vi "Top.vi"(8 "error in (no error)":errorcluster, 11 "Thread in":refnum<class "Thread.lvclass">) -> (0 "error":errorcluster, 3 "Thread out":refnum<class "Thread.lvclass">)   [LabVIEW 2017, in "DSF Core.lvlib" / "Thread.lvclass"]
uses:
  Thread.lvclass
  Thread State.ctl
  Thread.lvclass/Thread.ctl
  Thread Parameters/Thread Parameters.lvclass/Thread Parameters.ctl
  <vilib>/Platform/TimedLoop/XDataNode/timing_clust.ctl
  <vilib>/Platform/TimedLoop/XDataNode/nitl_modes.ctl
  <vilib>/Platform/TimedLoop/XDataNode/wakeup.ctl
  <vilib>/platform/TimedLoop/XDataNode/XDataNode.xnode
  <vilib>/Platform/TimedLoop/XDataNode/XDNodeRunTimeDep.lvlib
  Thread Parameters/Thread Parameters.lvclass
panel:
  out "Run Count":i32
  out "State":T1
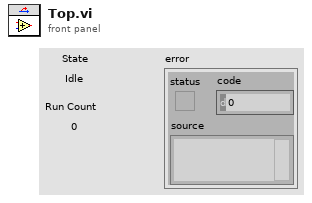
[diagram p1: front panel]
types:
  T1 = typedef "DSF Core.lvlib/Thread.lvclass/Thread State.ctl" = enum8{"Idle", "Running", "Error", "Shut Down"}
  T2 = typedef "XDNodeRunTimeDep.lvlib/timing_clust.ctl" = cluster{"Expected End [f-1]":u64, "Actual End [f-1]":u64, "Finished Late? [f-1]":bool, "Expected End [i-1]":u64, "Actual End [i-1]":u64, "Finished Late? [i-1]":bool, "Expected Start [i]":u64, "Actual Start [i]":u64, "Expected Start [f]":u64, "Actual Start [f]":u64, "Source Name":string, "Structure Name":string, "Period":i64, "Deadline":i64, "Offset":i64, "Start":i64, "Priority":i32, "Timeout":i32, "Mode":T3, "Wakeup Reason":T4, "Error":errorcluster, "Source Type":string, "Secondary Source Type":string, "Global End Time":u64, "Global Start Time":u64, "Frame Duration":u64, "Iteration Duration":u64, "Assigned CPU":i32, "I/O Scan Engine Mode":u32}
  T3 = typedef "XDNodeRunTimeDep.lvlib/nitl_modes.ctl" = enum32{"No Change", "Process missed periods, maintain original phase", "Discard missed periods, maintain original phase", "Process missed periods, ignore original phase", "Discard missed periods, ignore original phase"}
  T4 = typedef "XDNodeRunTimeDep.lvlib/wakeup.ctl" = enum32{"Normal", "Aborted", "Asynchronous wakeup", "Timing source error", "Timed loop error", "Timeout"}
  T5 = typedef "DSF Core.lvlib/Thread.lvclass/Thread Command.ctl" = enum8{"Run", "Shutdown"}
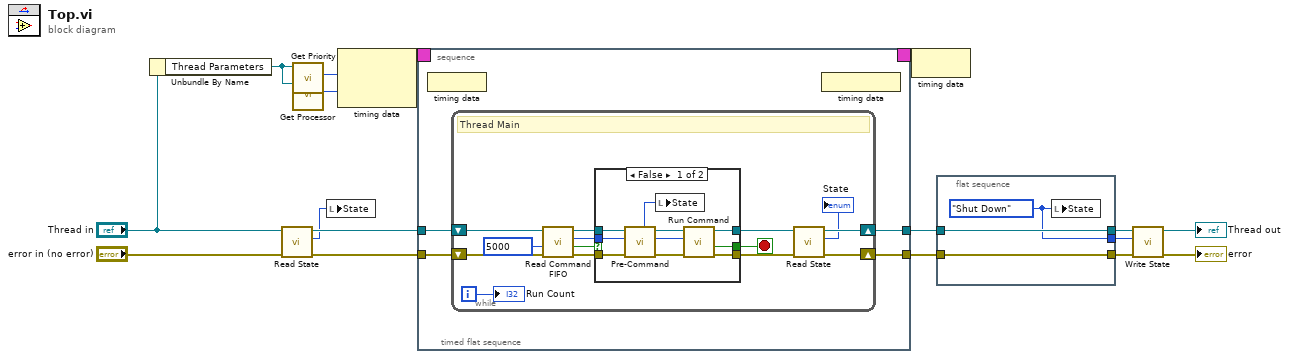
[diagram p0: block diagram]
diagram:
  n1 = Unbundle By Name("Thread in") -> ("Thread Parameters"=w13:refnum<class "Thread Parameters.lvclass">)
  n2 = call "Read State.vi"("error in (no error)"="error in (no error)", "Thread in"="Thread in") -> ("error out"=w4:errorcluster, "state"=w1:T1, "Thread out"=w5:refnum<class "Thread.lvclass">)  [unwired: 7 in]
  n3 = call "Get Priority.vi"("Thread Parameters in"=w13) -> ("Priority"=w12:i32)  [unwired: 9 in, 1 out]
  n4 = call "Get Processor.vi"("Thread Parameters in"=w13) -> ("Processor"=w11:i32)  [unwired: 9 in, 1 out]
  n5 = local write "State"(w1) -> ()
  n6 = node-c288(w12, w11) -> (w17:T2)
  n7 = timed-sequence {
    timing: w17 -> [_]
    timing-out: [_] -> w16
    tunnel: w4 -> [w21]
    tunnel: [w20] -> w8
    tunnel: [w19] -> w9
    tunnel: w5 -> [w18]
    n8 = timed-flat-sequence {
      tunnel: w21 -> [w22]
      tunnel: [w25] -> w20
      tunnel: [w24] -> w19
      tunnel: w18 -> [w23]
      n9 = node-c288() -> ()  [unwired: 1 in]
      n10 = while {
        shift-right: [w29] -> w24
        shift-left: w23 -> [w39]
        shift-right: [w28] -> w25
        shift-left: w22 -> [w32]
        i -> [w26]
        stop <- w33 stop-if-true
        # "Thread Main"
        n11 = call "Read Command FIFO.vi"("error in (no error)"=w32, "timeout in ms (0)"=5000, "Thread in"=w39) -> ("error out"=w37:errorcluster, "timed out?"=w34:bool, "command"=w36:T5, "Thread out"=w38:refnum<class "Thread.lvclass">)  [unwired: 4 in, 1 out]
        n12 = case shown="False" w34 {
          selector: w34 -> [_ w50]
          tunnel: [w49 w51] -> w30
          tunnel: [w48 w52] -> w31
          tunnel: w38 -> [w45 w52]
          tunnel: w37 -> [w46 w51]
          tunnel: w36 -> [w44 _]
          tunnel: [w47 w50] -> w33
          frame False {
            n13 = call "Pre-Command.vi"("error in (no error)"=w46, "command in"=w44, "Thread in"=w45) -> ("error out"=w41:errorcluster, "command out"=w43:T5, "Thread out"=w42:refnum<class "Thread.lvclass">, "state"=w40:T1)  [unwired: 5 in]
            n14 = local write "State"(w40) -> ()
            n15 = call "Run Command.vi"("error in (no error)"=w41, "command"=w43, "Thread in"=w42) -> ("error out"=w49:errorcluster, "shutdown?"=w47:bool, "Thread out"=w48:refnum<class "Thread.lvclass">)  [unwired: 6 in]
          }
          frame True {
          }
        }
        n16 = call "Read State.vi"("error in (no error)"=w30, "Thread in"=w31) -> ("error out"=w28:errorcluster, "state"=→"State":T1, "Thread out"=w29:refnum<class "Thread.lvclass">)  [unwired: 7 in]
        "Run Count" <- w26
      }
      n17 = node-c288() -> ()  [unwired: 1 out]
    }
  }
  n18 = node-c288(w16) -> ()
  n19 = flat-sequence {
    tunnel: [w55] -> w10
    tunnel: w9 -> [w56]
    tunnel: w8 -> [w57]
    tunnel: [w57] -> w7
    tunnel: [w56] -> w6
    frame #0 {
      w55 = Thread_State."Shut Down" ("state")
      n20 = local write "State"(w55) -> ()
    }
  }
  n21 = call "Write State.vi"("error in (no error)"=w7, "state"=w10, "Thread in"=w6) -> ("error out"=→"error":errorcluster, "Thread out"=→"Thread out":refnum<class "Thread.lvclass">)  [unwired: 7 in]
